vi "Test - CryptGenRandom.vi"() -> ()   [LabVIEW 2013]
uses:
  advapi32.dll
panel:
  out "Random Value (hexadecimal)":string
  out "Random Value (non-printable ASCII)":string
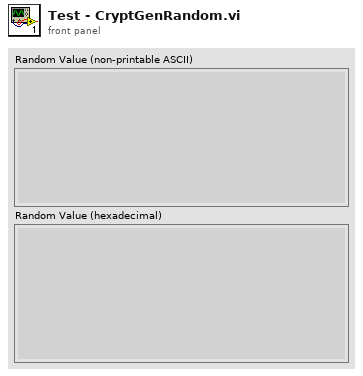
[diagram p1: front panel]
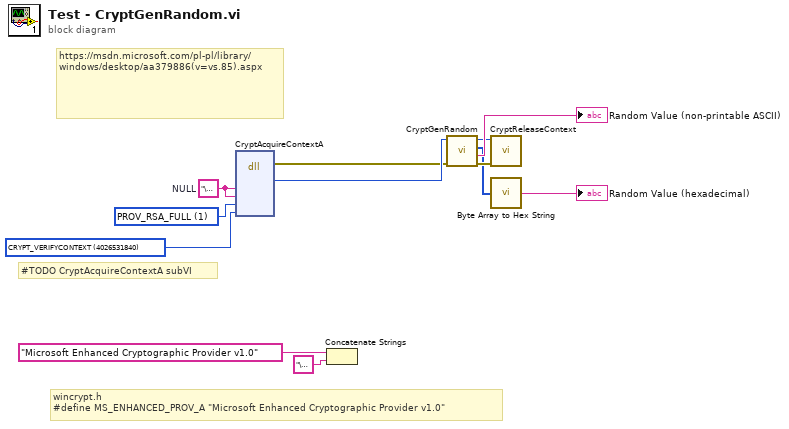
[diagram p0: block diagram]
diagram:
  w11 = u32 4026531840 items=["CRYPT_VERIFYCONTEXT"=4026531840, "CRYPT_NEWKEYSET"=8, "CRYPT_MACHINE_KEYSET"=32, "CRYPT_DELETEKEYSET"=16, "CRYPT_SILENT"=64, "CRYPT_DEFAULT_CONTAINER_OPTIONAL"=128]
  w12 = u32 1 items=["PROV_RSA_FULL"=1, "PROV_RSA_SIG"=2, "PROV_DSS"=3, "PROV_FORTEZZA"=4, "PROV_MS_EXCHANGE"=5, "PROV_SSL"=6, "PROV_RSA_SCHANNEL"=12, "PROV_DSS_DH"=13, "PROV_EC_ECDSA_SIG"=14, "PROV_EC_ECNRA_SIG"=15, "PROV_EC_ECDSA_FULL"=16, "PROV_EC_ECNRA_FULL"=17, "PROV_DH_SCHANNEL"=18, "PROV_SPYRUS_LYNKS"=20, "PROV_RNG"=21, "PROV_INTEL_SEC"=22, "PROV_REPLACE_OWF"=23, "PROV_RSA_AES"=24]
  w8 = "\u0000"  # NULL
  # "wincrypt.h\n#define MS_ENHANCED_PROV_A\t\"Microsoft Enhanced Cryptographic Provider v1.0\""
  # "#TODO CryptAcquireContextA subVI"
  # "https://msdn.microsoft.com/pl-pl/library/windows/desktop/aa379886(v=vs.85).aspx"
  n1 = dll-call lib="advapi32.dll" fn="CryptAcquireContextA"("pszContainer"=w8, "pszProvider"=w8, "dwProvType"=w12, "dwFlags"=w11) -> (error out=w3:errorcluster, "phProv"=w6:u32)  [unwired: 9 in, 1 out]
  n2 = Concatenate Strings("Microsoft Enhanced Cryptographic Provider v1.0", "\u0000" ("string")) -> ()  [unwired: 1 out]
  n3 = call "CryptGenRandom.vi"("error in (no error)"=w3, "CSP handle in"=w6) -> ("error out"=w4:errorcluster, "random bytes in hex"=→"Random Value (non-printable ASCII)":string, "random bytes array"=w2:u8[], "CSP handle out"=w5:u32)  [unwired: 5 in, 1 out]
  n4 = call "CryptReleaseContext.vi"("error in (no error)"=w4, "CSP handle in"=w5) -> ()  [unwired: 8 in, 2 out]
  n5 = call "Byte Array to Hex String.vi"("bytes array"=w2) -> ("hex string (normal display)"=→"Random Value (hexadecimal)":string)
